vi "MeasureRMS.vi"(8 "stop":bool, 9 "Sampling rate (Hz)":dbl, 10 "Number of Samples":dbl) -> (1 "RMS":dbl format="%0.2f", 2 "Waveform Graph":dynamicdata(graph))   [LabVIEW 2015]
uses:
  <vilib>/Analysis/NI_AALPro.lvlib
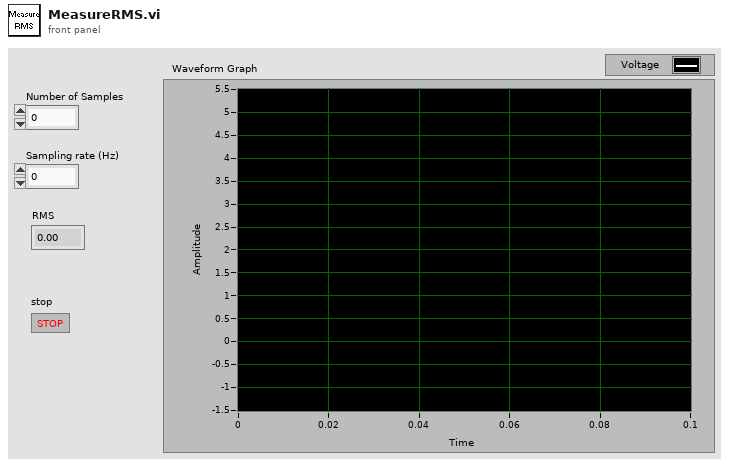
[diagram p1: front panel]
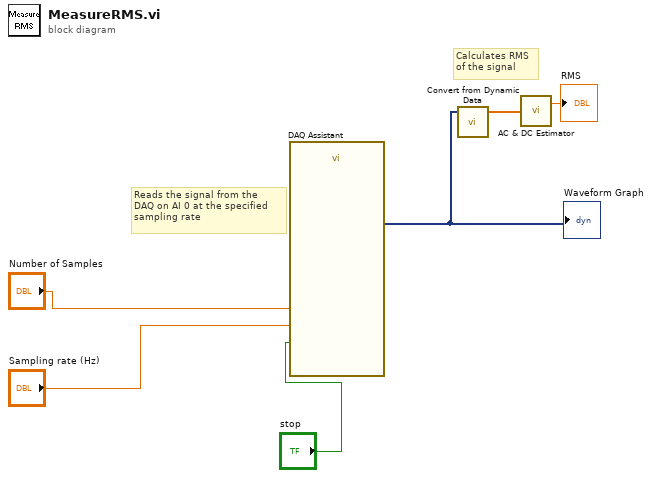
[diagram p0: block diagram]
diagram:
  # "Calculates RMS\nof the signal"
  # "Reads the signal from the \nDAQ on AI 0 at the specified \nsampling rate"
  n1 = call "DAQ Assistant"("rate"="Sampling rate (Hz)", "number of samples"="Number of Samples", "stop (T)"="stop") -> ("data"=w4:dynamicdata)  [unwired: 14 in, 2 out]
  "Waveform Graph" <- w4
  n2 = call "Convert from Dynamic Data"("Dynamic Data Type"=w4) -> ("Array"=w3:dbl[])  [unwired: 3 in]
  n3 = call <vilib>:"AC & DC Estimator.vi"("Signal (V)"=w3) -> ("AC estimate (Vrms)"=→"RMS":dbl)  [unwired: 1 out]
